vi "TFP LabVIEW GUI.vi"() -> ()   [LabVIEW 2010]
uses:
  <vilib>/Instr/_visa.llb/VISA Configure Serial Port (Instr).vi
panel:
  in  "?":bool
  in  "Move Right":bool
  in  "Move Left":bool
  in  "Rewind":bool
  in  "Taper":bool
  in  "?":refnum<visa-resource-name>="COM1"
  # "Arduino Configuration"
  # "Tapering Controls"
  # "Manual Alignment Controls"
  # "(C) Southern Methodist University\n2011 Senior Design\nPaul Coroneos and Rod Meikle"
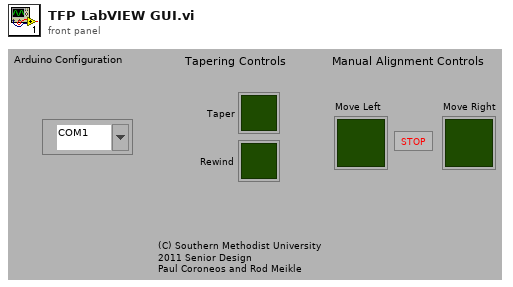
[diagram p1: front panel]
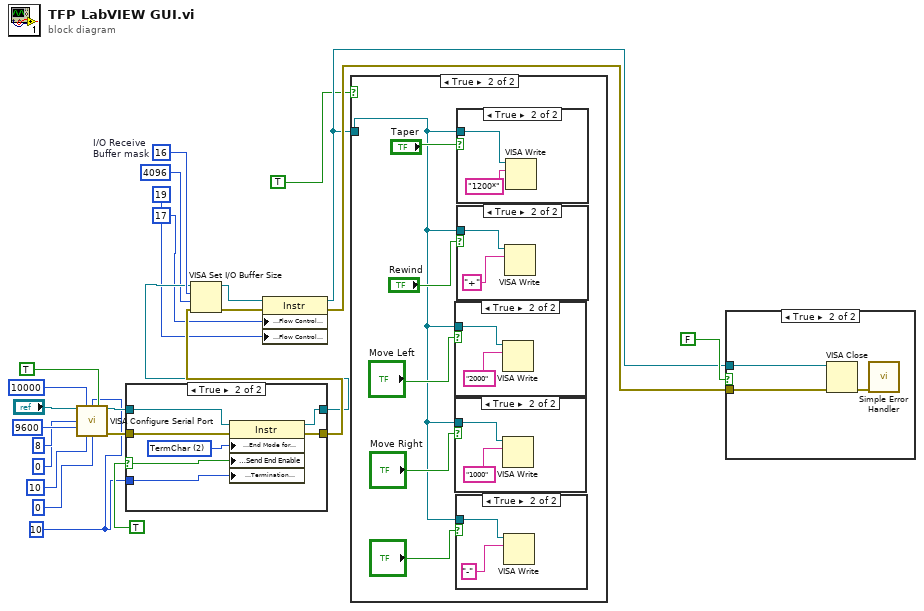
[diagram p0: block diagram]
diagram:
  w5 = u8 10
  w22 = u16 16  # I/O Receive Buffer mask
  n1 = call-poly "VISA Configure Serial Port"("VISA resource name"="?", "timeout (10sec)"=u32 10000, "termination char\n(0xA = '\\n' = LF)"=w5, "Enable Termination\nChar (T)"=TRUE, "baud rate (9600)"=u32 9600 ("Baud Rate"), "data bits (8)"=u16 8, "parity (0:none)"=u16 0, "stop bits (10: 1 bit)"=u16 10, "flow control (0:none)"=u16 0) -> ("VISA resource name out"=w16:refnum<visa-resource-name>, "error out"=w19:errorcluster)  [unwired: 1 in, 4 out]
  n2 = case shown="True" TRUE {
    selector: TRUE -> [_ w27]
    tunnel: w16 -> [w25 w33]
    tunnel: w19 -> [w26 w32]
    tunnel: [w25 w31] -> w17
    tunnel: [w26 w30] -> w18
    tunnel: w5 -> [_ w28]
    frame False {
    }
    frame True {
      w29 = u16 2 items=["None", "LastBit", "TermChar", "Break"] ("Serial Settings:Serial End Mode for Writes")
      n3 = property class="Instr"(reference=w33, error in=w32, "Serial Settings:End Mode for Writes"=w29, "Message Based Settings:Send End Enable"=w27, "Message Based Settings:Termination Character"=w28) -> (reference out=w31:refnum<visa-resource-name>, error out=w30:errorcluster)
    }
  }
  n4 = VISA Set I/O Buffer Size(VISA resource name=w17, mask (16)=w22, size (4096)=u32 4096, error in (no error)=w18) -> (VISA resource name out=w21:refnum<visa-resource-name>, error out=w20:errorcluster)
  n5 = property class="Instr"(reference=w21, error in=w20, "Serial Settings:Flow Control XON Character"=u8 17, "Serial Settings:Flow Control XOFF Character"=u8 19) -> (reference out=w2:refnum<visa-resource-name>, error out=w3:errorcluster)
  n6 = case shown="True" TRUE {
    tunnel: w2 -> [_ w34]
    frame False {
    }
    frame True {
      n7 = case shown="True" "Move Left" {
        tunnel: w34 -> [_ w44]
        frame False {
        }
        frame True {
          n8 = VISA Write(VISA resource name=w44, write buffer="2000") -> ()  [unwired: 1 in, 3 out]
        }
      }
      n9 = case shown="True" "Move Right" {
        tunnel: w34 -> [_ w42]
        frame False {
        }
        frame True {
          n10 = VISA Write(VISA resource name=w42, write buffer="1000") -> ()  [unwired: 1 in, 3 out]
        }
      }
      n11 = case shown="True" "?" {
        tunnel: w34 -> [_ w40]
        frame False {
        }
        frame True {
          n12 = VISA Write(VISA resource name=w40, write buffer="-") -> ()  [unwired: 1 in, 3 out]
        }
      }
      n13 = case shown="True" "Taper" {
        tunnel: w34 -> [_ w48]
        frame False {
        }
        frame True {
          n14 = VISA Write(VISA resource name=w48, write buffer="1200*") -> ()  [unwired: 1 in, 3 out]
        }
      }
      n15 = case shown="True" "Rewind" {
        tunnel: w34 -> [_ w46]
        frame False {
        }
        frame True {
          n16 = VISA Write(VISA resource name=w46, write buffer="+") -> ()  [unwired: 1 in, 3 out]
        }
      }
    }
  }
  n17 = case shown="True" FALSE {
    tunnel: w2 -> [_ w51]
    tunnel: w3 -> [_ w50]
    frame False {
    }
    frame True {
      n18 = VISA Close(VISA resource name=w51, error in (no error)=w50) -> (error out=w52:errorcluster)
      n19 = call <vilib>:"Simple Error Handler.vi"("error in (no error)"=w52) -> ()  [unwired: 1 in, 8 out]
    }
  }
